vi "tcs shm put Sample kernel Dawdle Filter LV.vi"(8 "error in (no error)":errorcluster, 11 "kernel_DawdleFilter_Ctl":cluster{"Bypass":i32, "T":sgl}) -> (0 "error out":errorcluster, 2 "function return":i32, 3 "kernel_DawdleFilter_Ctl out":cluster{"Bypass":i32, "T":sgl})   [LabVIEW 2016, in "SALLV_tcs.lvlib"]
doc: "int tcs_shm_putSample_kernel_DawdleFilterLV(tcs_kernel_DawdleFilterLV *kernel_DawdleFilter_Ctl );"
uses:
  SALLV_tcs.lvlib
  SALLV_tcs.so
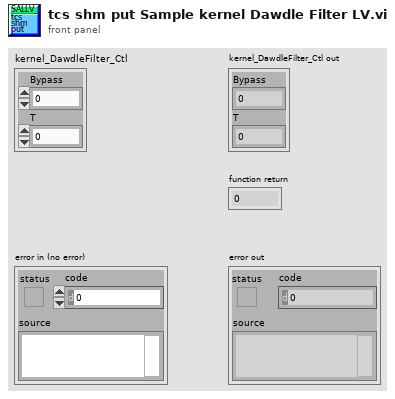
[diagram p1: front panel]
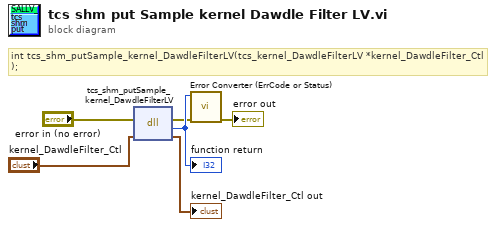
[diagram p0: block diagram]
diagram:
  # "int tcs_shm_putSample_kernel_DawdleFilterLV(tcs_kernel_DawdleFilterLV *kernel_DawdleFilter_Ctl );"
  n1 = dll-call lib="home/andres/Desktop/SALLV_tcs/SALLV_tcs.*" fn="tcs_shm_putSample_kernel_DawdleFilterLV"(error in="error in (no error)", "kernel_DawdleFilter_Ctl"="kernel_DawdleFilter_Ctl") -> (error out=w2:errorcluster, w6:i32, "kernel_DawdleFilter_Ctl"=→"kernel_DawdleFilter_Ctl out":cluster{"Bypass":i32, "T":sgl})  [unwired: 2 in, 1 out]
  "function return" <- w6
  n2 = call "Error Converter (ErrCode or Status).vi"("error in (no error)"=w2, "error code"=w6) -> ("error out"=→"error out":errorcluster)  [unwired: 9 in]
